vi "FV-resample-split_R140.vi"(5 "Max Frequency":dbl, 10 "R140":T1) -> (1 "Second Part":T1, 2 "First Part":T1)   [LabVIEW 2020, in "FV-file_viewer.lvlib"]
uses:
  FV-file_viewer.lvlib
  record_file_handler/VFH-file_cluster-R140.ctl
  record_file_handler/VFH-VNA_File_Handler.lvlib
panel:
  out "Frequency":dbl[](array[numeric])
  out "First Split":i32
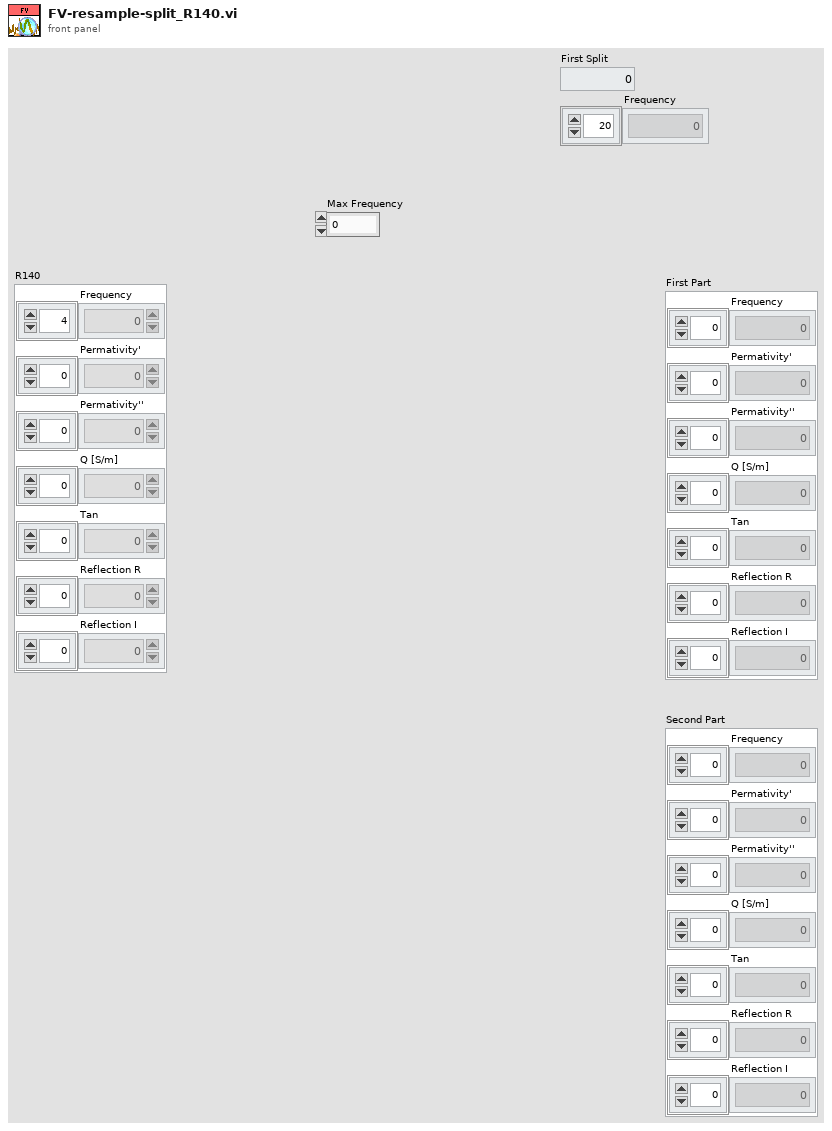
[diagram p1: front panel]
types:
  T1 = typedef "VFH-VNA_File_Handler.lvlib/VFH-file_cluster-R140.ctl" = cluster{"Frequency":dbl[], "Permativity'":dbl[], "Permativity''":dbl[], "Q [S/m]":dbl[], "Tan":dbl[], "Reflection R":dbl[], "Reflection I":dbl[]}
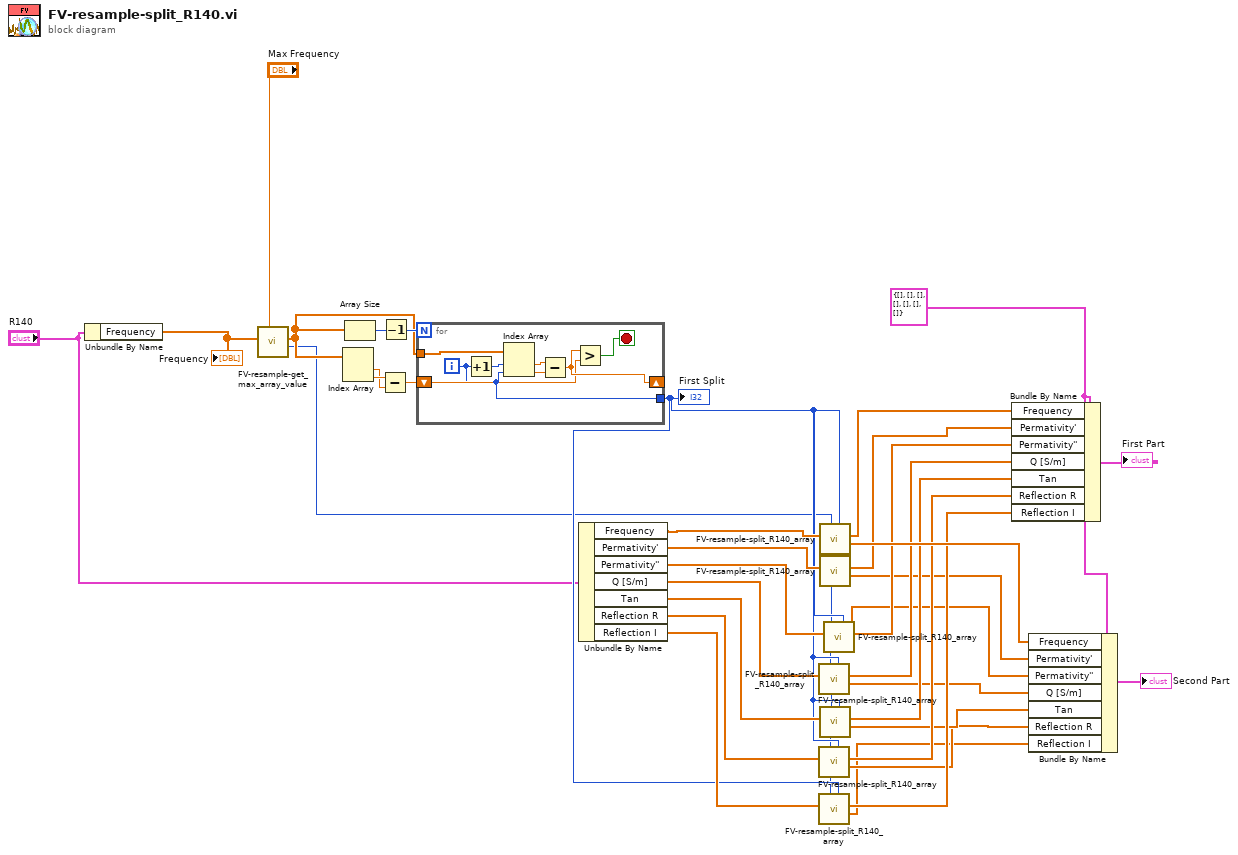
[diagram p0: block diagram]
diagram:
  w17 = T1 {"Frequency"=[], "Permativity'"=[], "Permativity''"=[], "Q [S/m]"=[], "Tan"=[], "Reflection R"=[], "Reflection I"=[]} ("First Part")
  n1 = Unbundle By Name("R140") -> ("Frequency"=w34:dbl[])
  "Frequency" <- w34
  n2 = call "FV-resample-get_max_array_value.vi"("max Frequency"="Max Frequency", "Frequency array"=w34) -> ("Position"=w18:i32, "cut array"=w28:dbl[])  [unwired: 8 in]
  n3 = Index Array(array=w28) -> (element #1=w32:dbl, element #2=w33:dbl)  [unwired: 2 in]
  n4 = Array Size(array=w28) -> (size(s)=w30:i32)
  n5 = Subtract(x=w33, y=w32) -> (x-y=w31:dbl)
  n6 = Decrement(x=w30) -> (x-1=w29:i32)
  n7 = for {
    N: w29 -> [_]
    tunnel: w28 -> [w43]
    shift-right: [w39] -> _
    shift-left: w31 -> [w38]
    tunnel: [w37] -> w19
    i -> [w37]
    stop <- w36 stop-if-true
    n8 = Increment(x=w37) -> (x+1=w42:i32)
    n9 = Index Array(array=w43, index #1=w42, index #2=w37) -> (element #1=w41:dbl, element #2=w40:dbl)
    n10 = Subtract(x=w41, y=w40) -> (x-y=w39:dbl)
    n11 = Greater?(x=w39, y=w38) -> (0:w36:bool)
  }
  "First Split" <- w19
  n12 = Unbundle By Name("R140") -> ("Frequency"=w27:dbl[], "Permativity'"=w25:dbl[], "Permativity''"=w24:dbl[], "Q [S/m]"=w23:dbl[], "Tan"=w22:dbl[], "Reflection R"=w21:dbl[], "Reflection I"=w20:dbl[])
  n13 = call "FV-resample-split_R140_array.vi"("Mid split"=w19, "First split"=w18, "double array"=w23) -> ("second subarray"=w5:dbl[], "first subarray"=w11:dbl[])  [unwired: 7 in]
  n14 = call "FV-resample-split_R140_array.vi"("Mid split"=w19, "First split"=w18, "double array"=w21) -> ("second subarray"=w3:dbl[], "first subarray"=w9:dbl[])  [unwired: 7 in]
  n15 = call "FV-resample-split_R140_array.vi"("Mid split"=w19, "First split"=w18, "double array"=w20) -> ("second subarray"=w2:dbl[], "first subarray"=w8:dbl[])  [unwired: 7 in]
  n16 = call "FV-resample-split_R140_array.vi"("Mid split"=w19, "First split"=w18, "double array"=w27) -> ("second subarray"=w14:dbl[], "first subarray"=w15:dbl[])  [unwired: 7 in]
  n17 = call "FV-resample-split_R140_array.vi"("Mid split"=w19, "First split"=w18, "double array"=w25) -> ("second subarray"=w7:dbl[], "first subarray"=w13:dbl[])  [unwired: 7 in]
  n18 = call "FV-resample-split_R140_array.vi"("Mid split"=w19, "First split"=w18, "double array"=w22) -> ("second subarray"=w4:dbl[], "first subarray"=w10:dbl[])  [unwired: 7 in]
  n19 = call "FV-resample-split_R140_array.vi"("Mid split"=w19, "First split"=w18, "double array"=w24) -> ("second subarray"=w6:dbl[], "first subarray"=w12:dbl[])  [unwired: 7 in]
  n20 = Bundle By Name(cluster=w17, "Frequency"=w15, "Permativity'"=w13, "Permativity''"=w12, "Q [S/m]"=w11, "Tan"=w10, "Reflection R"=w9, "Reflection I"=w8) -> (→"First Part":T1)
  n21 = Bundle By Name(cluster=w17, "Frequency"=w14, "Permativity'"=w7, "Permativity''"=w6, "Q [S/m]"=w5, "Tan"=w4, "Reflection R"=w3, "Reflection I"=w2) -> (→"Second Part":T1)
